vi "Union Unified Msg Set.vi"(11 "TEMPLATE Actor in":refnum<class "TEMPLATE Actor.lvclass">) -> (2 "Unified Msg Set":T1)   [LabVIEW 2025, in "_Template.lvlib" / "Templates.lvlib" / "TEMPLATE Actor.lvlib" / "TEMPLATE Actor.lvclass"]
uses:
  TEMPLATE Actor.lvclass
  C:/git/jettl/src/jettl/jettl/Actor/Actor.lvclass
  jettl/jettl/Msg Set.ctl
  jettl/jettl/Msg/Msg.lvclass
  jettl/jettl/Actor/Actor.lvclass
  TEMPLATE Actor.lvclass/TEMPLATE Actor.ctl
  jettl/jettl/jettl.lvlib
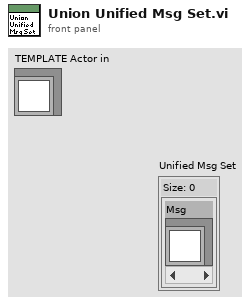
[diagram p1: front panel]
types:
  T1 = typedef "jettl.lvlib/Msg Set.ctl" = set{refnum<class "Msg.lvclass">}
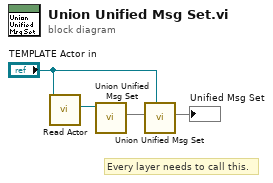
[diagram p0: block diagram]
diagram:
  # "Every layer needs to call this."
  n1 = call-dynamic "Read Actor.vi"("TEMPLATE Actor in"="TEMPLATE Actor in") -> ("Actor"=w2:refnum<class "Actor.lvclass">)  [unwired: 10 in]
  n2 = call-dynamic "Union Unified Msg Set.vi"("Get Actor in"=w2) -> ("Unified Msg Set"=w1:T1)  [unwired: 10 in]
  n3 = call "Union Unified Msg Set.vi"("Actor"="TEMPLATE Actor in", "Unified Msg Set in"=w1) -> ("Unified Msg Set out"=→"Unified Msg Set":T1)  [unwired: 9 in]
